vi "Waveform Inputs.vi"(8 "error in (no error)":errorcluster, 11 "Node Ptr":T1 format="%.0x") -> (0 "error out":errorcluster)   [LabVIEW 2019, in "FPGA Addon System Explorer.lvlib"]
uses:
  FPGA Addon System Explorer.lvlib
  <vilib>/NI VeriStand/Custom Device API/Custom Device Item Ref.ctl
  Addon Shared/Types/FG Action.ctl
  Types/Channel Type.ctl
  Addon Shared/SubVIs/Constants.vi
  <vilib>/NI/NI VeriStand Advanced SysDef API/SysDef API/SysDef.Property.Get.vi
  <vilib>/NI/NI VeriStand Advanced SysDef API/_SubVIs/SysDef.Property.Get.Variant.vi
  <vilib>/NI/NI VeriStand Advanced SysDef API/SysDef API/SysDef.Property.Set.vi
  <vilib>/NI/NI VeriStand Advanced SysDef API/_SubVIs/SysDef.Property.Set.Variant.vi
  <vilib>/NI VeriStand/Custom Device API/Custom Device API.lvlib
  Addon Shared/FPGA Addon Shared.lvlib
panel:
  in  "remove":bool
  in  "add":bool
  in  "Available DMA":i32[](listbox)
  in  "Header 2":cluster{"Section Name":string}={"Section Name"="Custom Device Item Settings"}
  in  "SHDocVw.IWebBrowser":refnum<k7>(container)
  in  "Header":cluster{"Section Name":string}={"Section Name"="Custom Device Item Settings"}
  in  "Description":string
  out "Name":string
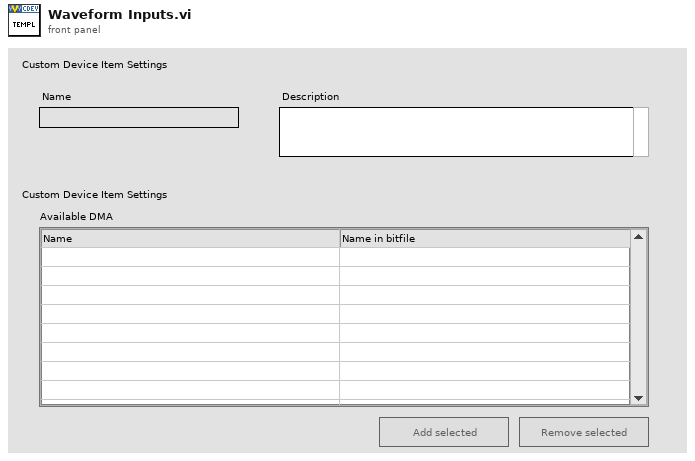
[diagram p1: front panel]
types:
  T1 = typedef "Custom Device API.lvlib/Custom Device Item Ref.ctl" = u64
  T2 = typedef "FPGA Addon Shared.lvlib/FG Action.ctl" = enum8{"GET", "SET"}
  T3 = typedef "Custom Device API.lvlib/Custom Device Item Info.ctl" = cluster{"Name":string, "Is Channel":bool, "GUID":string, "Is Waveform":bool}
  T4 = typedef "FPGA Addon Shared.lvlib/DMA Information.ctl" = cluster{"Name":string, "Data Type":T5}
  T5 = typedef "FPGA Addon Shared.lvlib/Data Type.ctl" = enum8{"<Null>", "I8", "I16", "I32", "I64", "U8", "U16", "U32", "U64", "SGL", "Boolean", "Analog PWM In Settings", "Analog PWM In", "Digital PWM In Settings", "Digital PWM In", "Digital PWM Out", "Sine Out", "FXP+/-24.5", "FXP+/-16.5", "FXP+/-32.8", "FXP+/-64.32", "FXP+/-16.7", "FXP+/-20.5", "FXP+/-27.5", "FXP+/-32.16", "FXP +16.3", "FXP +18.3", "Digital Static In", "Digital Static Out", "Digital Static In Settings", "Digital WSS Out", "Quad Encoder Settings", "Quad Encoder In"}
  T6 = typedef "FPGA Addon System Explorer.lvlib/Listbox Cluster.ctl" = cluster{"add":refnum<vi>, "remove":refnum<vi>, "Listbox":refnum<vi>, "selected":i32[], "not present":i32[], "listbox text":string[][], "Section Ref":T1}
  T7 = typedef "FPGA Addon System Explorer.lvlib/Channel Type.ctl" = enum16{"Write Channel", "Read Channel", "Write Waveform", "Read Waveform"}
  T8 = typedef "Custom Device API.lvlib/Custom Device Commands.ctl" = enum16{"Default", "Item renamed", "Shutdown", "Dynamic button pressed"}
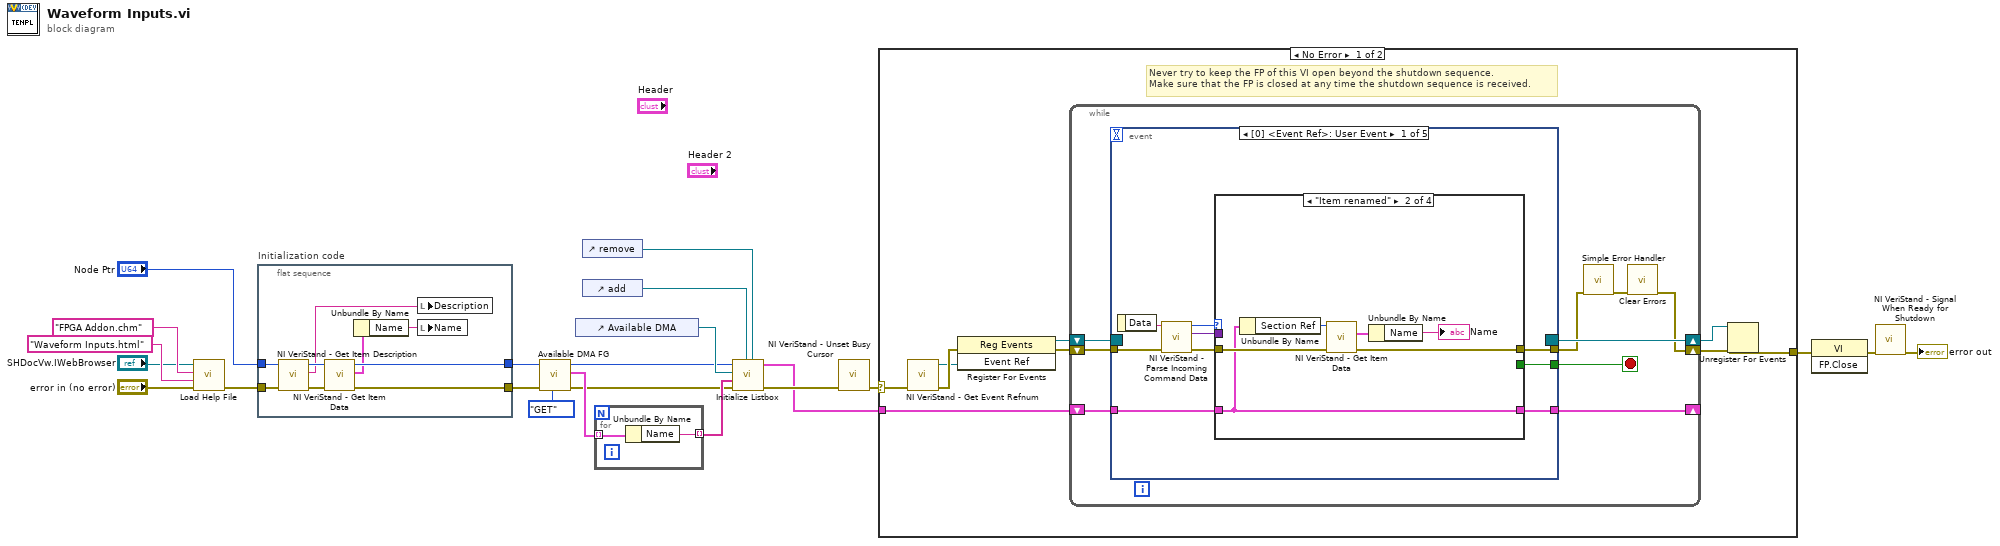
[diagram p0: block diagram]
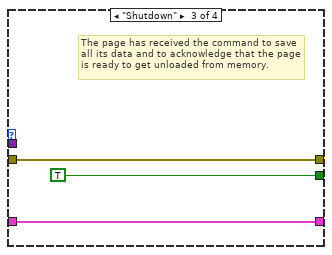
[diagram p3: hidden frame]
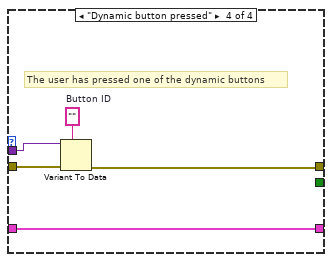
[diagram p4: hidden frame]
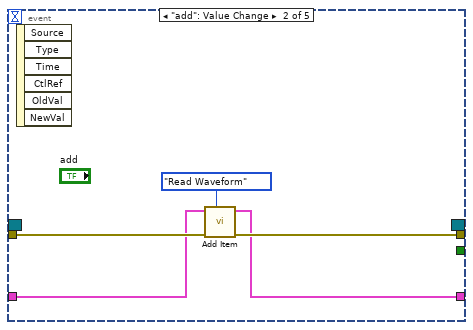
[diagram p5: hidden frame]
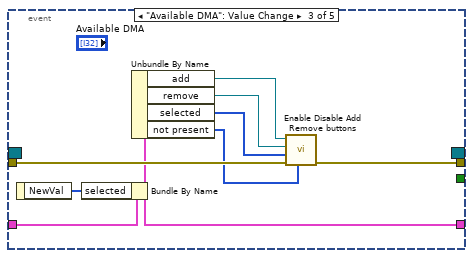
[diagram p6: hidden frame]
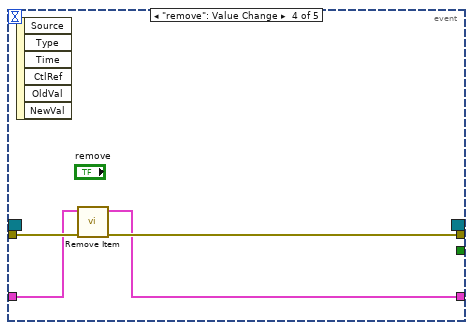
[diagram p7: hidden frame]
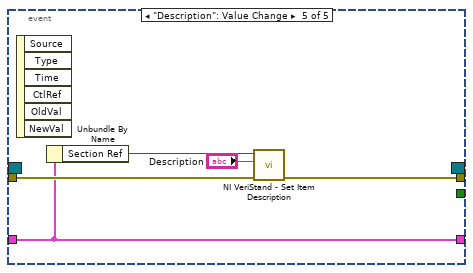
[diagram p8: hidden frame]
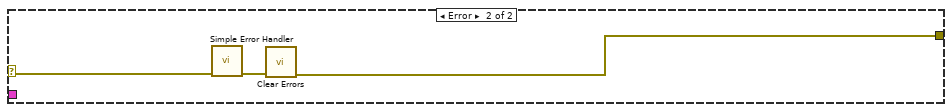
[diagram p9: hidden frame]
diagram:
  n1 = call "Load Help File.vi"("error in (no error)"="error in (no error)", "HTML File"="Waveform Inputs.html", "Main CHM File"="FPGA Addon.chm", "SHDocVw.IWebBrowser2"="SHDocVw.IWebBrowser") -> ("error out"=w17:errorcluster)  [unwired: 7 in]
  n2 = flat-sequence "Initialization code" {
    tunnel: w17 -> [w29]
    tunnel: "Node Ptr" -> [w28]
    tunnel: [w23] -> w2
    tunnel: [w31] -> w6
    frame #0 {
      n3 = call <vilib>:"NI VeriStand - Get Item Description.vi"("error in (no error)"=w29, "Item Ref in"=w28) -> ("error out"=w26:errorcluster, "Description"=w27:string, "Item Ref out"=w30:T1)  [unwired: 7 out]
      n4 = call <vilib>:"NI VeriStand - Get Item Data.vi"("error in (no error)"=w26, "Item Ref in"=w30) -> ("error out"=w23:errorcluster, "Item Info"=w25:T3, "Item Ref out"=w31:T1)  [unwired: 7 out]
      n5 = Unbundle By Name(w25) -> ("Name"=w24:string)
      n6 = local write "Description"(w27) -> ()
      n7 = local write "Name"(w24) -> ()
    }
  }
  n8 = call "Available DMA FG.vi"("Action"=FG_Action."GET", "error in (no error)"=w2, "Item Ref"=w6) -> ("error out"=w1:errorcluster, "Available DMA"=w4:T4[], "Item Ref out"=w5:T1)  [unwired: 6 in]
  n9 = control-ref of="Available DMA"() -> (w11:refnum<vi>)
  n10 = control-ref of="remove"() -> (w14:refnum<vi>)
  n11 = control-ref of="add"() -> (w15:refnum<vi>)
  n12 = for {
    tunnel: w4 -> [w33] mode=indexing
    tunnel: [w32] -> w16 mode=indexing
    n13 = Unbundle By Name(w33) -> ("Name"=w32:string)
  }
  n14 = call "Initialize Listbox.vi"("remove"=w14, "add"=w15, "error in (no error)"=w1, "Names"=w16, "Listbox"=w11, "Item Ref"=w5) -> ("error out"=w13:errorcluster, "Listbox Refs"=w12:T6)  [unwired: 4 in]
  n15 = call <vilib>:"NI VeriStand - Unset Busy Cursor.vi"("error in (no error)"=w13) -> ("error out"=w20:errorcluster)  [unwired: 10 out]
  n16 = case shown="No Error" w20 {
    selector: w20 -> [w35 w102]
    tunnel: [w39 w100] -> w22
    tunnel: w12 -> [w34 _]
    frame No Error {
      # "Never try to keep the FP of this VI open beyond the shutdown sequence.\nMake sure that the FP is closed at any time the shutdown sequence is received."
      n17 = call <vilib>:"NI VeriStand - Get Event Refnum.vi"("error in (no error)"=w35) -> ("error out"=w42:errorcluster, "Event Ref"=w38:refnum<user-event>)  [unwired: 9 out]
      n18 = register-events(error in=w42, w38) -> (reference out=w36:refnum<event-registration>, error out=w37:errorcluster)  [unwired: 1 in]
      n19 = while {
        shift-right: [w45] -> w40
        shift-left: w37 -> [w50]
        shift-right: [w51] -> w41
        shift-left: w36 -> [w49]
        shift-right: [w43] -> _
        shift-left: w34 -> [w44]
        stop <- w48 stop-if-true
        n20 = event shown="[0] <Event Ref>: User Event" {
          selector: w49 -> [_ _ _ _ _]
          dyn-events: [_ _ _ _ _] -> w51
          timeout: _ -> [_ _ _ _ _]
          tunnel: w50 -> [w60 w81 w90 w93 w99]
          tunnel: [w56 _ _ _ _] -> w48
          tunnel: [w55 w80 w89 w94 w98] -> w47
          tunnel: w44 -> [w53 w78 w87 w92 w97]
          tunnel: [w52 w79 w86 w91 w97] -> w43
          event User Event {
            n21 = event-data() -> ("Data"=w59:string)  [unwired: 1 out]
            n22 = call <vilib>:"NI VeriStand - Parse Incoming Command Data.vi"("error in (no error)"=w60, "Incoming data"=w59) -> ("error out"=w58:errorcluster, "Outgoing data"=w54:variant, "Action"=w57:T8)  [unwired: 7 out]
            n23 = case shown="\"Item renamed\"" w57 {
              tunnel: w58 -> [w62 w68 w70 w76]
              tunnel: [_ _ TRUE _] -> w56
              tunnel: [w62 w66 w70 w73] -> w55
              tunnel: w54 -> [_ _ _ w75]
              tunnel: w53 -> [w61 w64 w69 w72]
              tunnel: [w61 w64 w69 w72] -> w52
              frame "Default", Default {
              }
              frame "Item renamed" {
                n24 = Unbundle By Name(w64) -> ("Section Ref"=w65:T1)
                n25 = call <vilib>:"NI VeriStand - Get Item Data.vi"("error in (no error)"=w68, "Item Ref in"=w65) -> ("error out"=w66:errorcluster, "Item Info"=w67:T3)  [unwired: 8 out]
                n26 = Unbundle By Name(w67) -> ("Name"=→"Name":string)
              }
              frame "Shutdown" {
                # "The page has received the command to save all its data and to acknowledge that the page is ready to get unloaded from memory."
              }
              frame "Dynamic button pressed" {
                w74 = ""  # Button ID
                # "The user has pressed one of the dynamic buttons"
                n27 = Variant To Data(error in=w76, type=w74, Variant=w75) -> (error out=w73:errorcluster)  [unwired: 1 out]
              }
            }
          }
          event "add": Value Change {
            n28 = event-data() -> ()  [unwired: 7 out]
            n29 = call "Add Item.vi"("Action"=Channel_Type."Read Waveform", "error in (no error)"=w81, "Listbox Refs in"=w78) -> ("error out"=w80:errorcluster, "Listbox Refs out"=w79:T6)  [unwired: 7 in]
          }
          event "Available DMA": Value Change {
            n30 = event-data() -> ("NewVal"=w85:i32[])  [unwired: 1 out]
            n31 = Bundle By Name(cluster=w87, "selected"=w85) -> (w86:T6)
            n32 = Unbundle By Name(w86) -> ("add"=w82:refnum<vi>, "remove"=w83:refnum<vi>, "selected"=w84:i32[], "not present"=w88:i32[])
            n33 = call "Enable Disable Add Remove buttons.vi"("not present item indexes"=w88, "error in (no error)"=w90, "selected items"=w84, "remove button"=w83, "add button"=w82) -> ("error out"=w89:errorcluster)  [unwired: 6 in]
          }
          event "remove": Value Change {
            n34 = event-data() -> ()  [unwired: 7 out]
            n35 = call "Remove Item.vi"("error in (no error)"=w93, "Listbox Refs in"=w92) -> ("error out"=w94:errorcluster, "Listbox Refs out"=w91:T6)  [unwired: 8 in]
          }
          event "Description": Value Change {
            n36 = event-data() -> ()  [unwired: 7 out]
            n37 = Unbundle By Name(w97) -> ("Section Ref"=w96:T1)
            n38 = call <vilib>:"NI VeriStand - Set Item Description.vi"("error in (no error)"=w99, "Description"="Description", "Item Ref in"=w96) -> ("error out"=w98:errorcluster)  [unwired: 8 out]
          }
        }
        n39 = call <vilib>:"Simple Error Handler.vi"("error in (no error)"=w47) -> ("error out"=w46:errorcluster)  [unwired: 1 in, 7 out]
        n40 = call <vilib>:"Clear Errors.vi"("error in (no error)"=w46) -> ("error out"=w45:errorcluster)  [unwired: 1 in, 5 out]
      }
      n41 = Unregister For Events(event registration refnum=w41, error in=w40) -> (error out=w39:errorcluster)
    }
    frame Error {
      n42 = call <vilib>:"Simple Error Handler.vi"("error in (no error)"=w102) -> ("error out"=w101:errorcluster)  [unwired: 1 in, 7 out]
      n43 = call <vilib>:"Clear Errors.vi"("error in (no error)"=w101) -> ("error out"=w100:errorcluster)  [unwired: 1 in, 5 out]
    }
  }
  n44 = invoke class="VI" method="FP.Close"(error in=w22) -> (error out=w21:errorcluster)  [unwired: 2 in, 2 out]
  n45 = call <vilib>:"NI VeriStand - Signal When Ready for Shutdown.vi"("error in (no error)"=w21) -> ("error out"=→"error out":errorcluster)  [unwired: 10 out]
